vi "1_Face_Detection_Model_Converter.vi"() -> ()   [LabVIEW 2020]
doc: "This example demonstrates the preparation process of pretrained Face Detection model to be deployed on FPGA.\nIt consists of the following stages:\n1. Network optimization by merging applicable layers together.\n2. Per layer weights and output statistics calculation for optimal quantization on FPGA.\n3. Saving converted model together with statistical information to be used during the deployment.\n\nMore Examples: https://github.com/ngenehub/deepltk_fpga_examples"
uses:
  <vilib>/Ngene/DeepLTK FPGA Addon/Toolkit/NNF_Host/Low_Level/Network_Converter/Controls/Range_Calculation_Specs.ctl
  <vilib>/Ngene/Deep Learning Toolkit/Toolkit/Deep_Learning_Toolkit_by_Ngene.lvlib
  <vilib>/Ngene/DeepLTK FPGA Addon/Toolkit/DeepLTK_FPGA_Addon.lvlib
panel:
  in  "Dataset Path (Images)":path
  out "error out":errorcluster
  in  "Wights file":path
  in  "Configuration file":path
  out "Generated_Files":path[](array[path])
  in  "Dest":path
  # "Overview: This example demonstrates the preparation process of pretrained Face Detection model to be deployed on FPGA.\nIt consists of the following stages:\n1. Network optimization by merging applicable layers together.\n2. Per layer weights and output statistics calculation for optimal quantization on FPGA.\n3. Saving converted model together with statistical information to be used during the deployment.\nRequirements:\n•DeepLTK - Deep Learning Toolkit for LabVIEW\n•DeepLTK FPGA Addon\n•Sample dataset for reliable output statistic calculation.\n•NI Vision Development Module\nInstructions: \nNote: This VI can run as is by automatically retrieving required files from the example. I.e. steps 1. - 2. are optional.\n1.\tProvide the path to the configuration file of a pretrained model in the \"Configuration File\" control.\n2.\tProvide the path to the weights file of a pretrained model in the \"Weights File\" control. \n3.\tProvide the path to the WIDER FACE dataset images in the \"Dataset Path (Images)\" control. Dataset link: http://shuoyang1213.me/WIDERFACE/ \n4.\tProvide the destination directory where the result will be stored in the \"Dest\" control.\n5.\tRun the VI and wait until all processes are completed.\n\nThe resulting files (Scalers .cfg, Weights .bin, and Configuration .cfg) will be stored at paths displayed in \"Generated_Files\" indicator.\nThis files will be used during inference process.\nMore Examples: https://github.com/ngenehub/deepltk_fpga_examples"
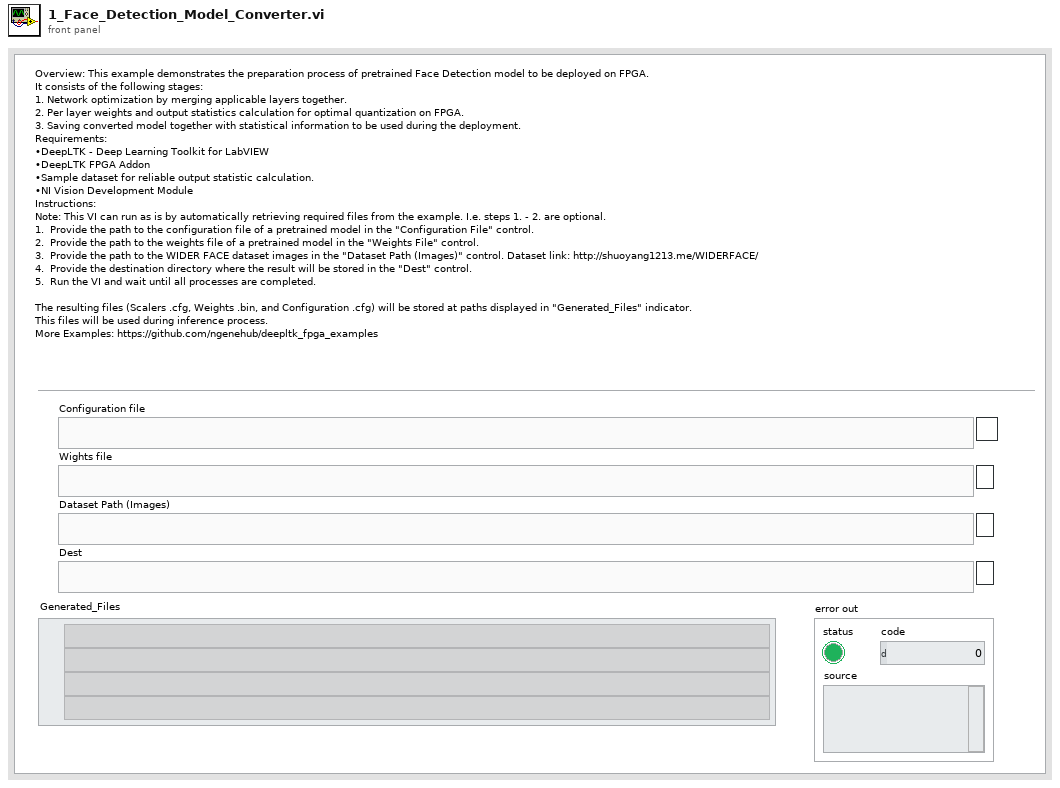
[diagram p1: front panel]
types:
  T1 = typedef "DeepLTK_FPGA_Addon.lvlib/Range_Calculation_Specs.ctl" = cluster{"# of Histogram Bins":i32, "Outputs Range Percentile(0.9999)":dbl, "Weights Range Percentile(0.9999)":dbl}
  T2 = typedef "Deep_Learning_Toolkit_by_Ngene.lvlib/NN_DataSet(In3D_OutBBox).ctl" = cluster{"Inputs Ref.":variant, "Dataset_Size":i32, "Dims_In":T3, "Outputs Refs":T4, "No of Classes ":i32, "Labels":string[], "File Paths":path[]}
  T3 = typedef "Deep_Learning_Toolkit_by_Ngene.lvlib/NN_Dims(C,H,W).ctl" = cluster{"C":i32, "H":i32, "W":i32}
  T4 = typedef "Deep_Learning_Toolkit_by_Ngene.lvlib/NN_Data_ref(1D_BBox).ctl" = refnum<data-value>
  T5 = typedef "Deep_Learning_Toolkit_by_Ngene.lvlib/NN_Config_Params.ctl" = cluster{"Name":string, "mBatch":i32, "NN_Train_Params":T6, "LR_Decay_Policy":T9, "Labels":string[], "Loss":T11}
  T6 = typedef "Deep_Learning_Toolkit_by_Ngene.lvlib/NN_Train_Params.ctl" = cluster{"Optimizer":T7, "Beta_1":sgl, "Beta_2":sgl, "Weight Decay(L1)":sgl, "Weight Decay(L2)":sgl, "Data_Sampling":T8}
  T7 = typedef "Deep_Learning_Toolkit_by_Ngene.lvlib/NN_Train_Optimizer.ctl" = enum16{"SGD", "Adam", "Adagrad", "Adadelta", "RMSProp", "Nesterov"}
  T8 = typedef "Deep_Learning_Toolkit_by_Ngene.lvlib/NN_Train_Data_Sampling.ctl" = enum16{"Random", "Sequential"}
  T9 = typedef "Deep_Learning_Toolkit_by_Ngene.lvlib/NN_LR_Policy_Cfg.ctl" = cluster{"Policy_Type":T10, "LR0":dbl, "k":sgl, "WarmUp_Policy":enum16{"Step", "Ramp"}, "WarmUp_Iter":i32, "WarmUp_Ratio":sgl}
  T10 = typedef "Deep_Learning_Toolkit_by_Ngene.lvlib/NN_LR_Policy_Type.ctl" = enum16{"Manual", "Step", "Exp", "1/t"}
  T11 = typedef "Deep_Learning_Toolkit_by_Ngene.lvlib/NN_Loss_Config_Params.ctl" = cluster{"Loss_Type":T12, "Loss_Conf_Params":variant}
  T12 = typedef "Deep_Learning_Toolkit_by_Ngene.lvlib/NN_Loss_Type.ctl" = enum16{"None", "MSE", "CrossEntropy", "YOLO_v2", "YOLO_v4"}
  T13 = typedef "Deep_Learning_Toolkit_by_Ngene.lvlib/NN_Layer_Config_Params.ctl" = cluster{"Layer_Type":T14, "Layer_Conf_Params":variant, "Input Layers":string[]}
  T14 = typedef "Deep_Learning_Toolkit_by_Ngene.lvlib/NN_Layer_Type.ctl" = enum16{"Input1D", "Input3D", "Conv1D", "Conv2D", "Conv2D_Adv", "MaxPool", "AvgPool", "UpSample", "DropOut3D", "ShortCut", "Concat", "SoftMax3D", "FC", "DropOut", "Softmax", "Flatten", "YOLO_v2", "YOLO_v4", "Activation", "BatchNormalization", "Unsupported"}
  T15 = typedef "Deep_Learning_Toolkit_by_Ngene.lvlib/NN.ctl" = cluster{"Name":string, "No of Layers":i32, "mBatch":i32, "Layers":T16[], "Dimty":T17, "Dims_In":T3, "Dims_Out":T3, "Working_Dir":path, "Train?":bool, "Train_Params":T6, "LR_Update_Policy":T9, "Session Data":T18, "Ground_truth":T19, "NNg_hdls":T20, "NN_Device":T21, "GPU Id":i32, "Labels":string[], "Receptive Field":T22[], "Loss_Type":T12, "Loss_Cfg_Prms":variant, "NNG_WS":T23}
  T16 = typedef "Deep_Learning_Toolkit_by_Ngene.lvlib/NN_Layer_ref.ctl" = refnum<data-value>
  T17 = typedef "Deep_Learning_Toolkit_by_Ngene.lvlib/NN_In_Out_Dim-ty.ctl" = enum8{"In1D_Out1D", "In3D_Out1D", "In3D_Out3D", "In3D_OutBBox"}
  T18 = typedef "Deep_Learning_Toolkit_by_Ngene.lvlib/NN_Train_Session_Data.ctl" = cluster{"Epochs":sgl, "Tot_Iter":i32, "LR":sgl, "LR_iter":i32}
  T19 = typedef "Deep_Learning_Toolkit_by_Ngene.lvlib/NN_Ground_truth.ctl" = cluster{"Y":variant}
  T20 = typedef "Deep_Learning_Toolkit_by_Ngene.lvlib/nng_cuda_handles.ctl" = cluster{"cudnn":u64, "cublas":u64, "stream":u64, "curand":u64}
  T21 = typedef "Deep_Learning_Toolkit_by_Ngene.lvlib/NN_Device.ctl" = enum16{"CPU", "GPU"}
  T22 = typedef "Deep_Learning_Toolkit_by_Ngene.lvlib/NN_Dims(V,H).ctl" = cluster{"V":i32, "H":i32}
  T23 = typedef "Deep_Learning_Toolkit_by_Ngene.lvlib/NNG_WS.ctl" = cluster{"NNG_WS_Mem":T24, "Max_WS_Size":i64}
  T24 = typedef "Deep_Learning_Toolkit_by_Ngene.lvlib/NNg_WS_Mem_DVR.ctl" = refnum<data-value>
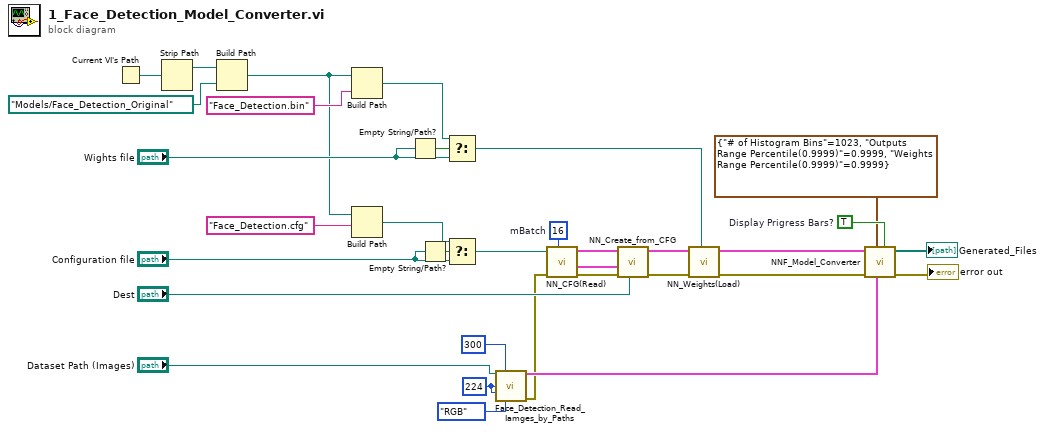
[diagram p0: block diagram]
diagram:
  w14 = 224 ("Img Height")
  w23 = TRUE  # Display Prigress Bars?
  w27 = 16  # mBatch
  n1 = Current VI's Path() -> (path=w4:path)
  n2 = Strip Path(path=w4) -> (stripped path=w6:path)  [unwired: 1 out]
  n3 = Build Path(base path=w6, name or relative path=path "Models/Face_Detection_Original" ("stripped path")) -> (appended path=w3:path)
  n4 = Build Path(base path=w3, name or relative path="Face_Detection.bin") -> (appended path=w2:path)
  n5 = Build Path(base path=w3, name or relative path="Face_Detection.cfg") -> (appended path=w1:path)
  n6 = Empty String/Path?(string/path="Wights file") -> (empty?=w15:bool)
  n7 = Empty String/Path?(string/path="Configuration file") -> (empty?=w16:bool)
  n8 = Select(t=w2, s=w15, f="Wights file") -> (s? t:f=w19:path)
  n9 = Select(t=w1, s=w16, f="Configuration file") -> (s? t:f=w20:path)
  n10 = call "Face_Detection_Read_Iamges_by_Paths.vi"("Dataset Path (Images)"="Dataset Path (Images)", "Max Sample count"=300, "Img Height"=w14, "Img Width"=w14, "Img Type"=enum16{"Grayscale", "RGB"}."RGB") -> ("NN_DataSet(In3D_OutBBox)"=w11:T2, "error out"=w10:errorcluster)  [unwired: 9 in]
  n11 = call <vilib>:"NN_CFG(Read).vi"("mBatch"=w27, "error in (no error)"=w10, "CFG file path"=w20) -> ("error out"=w30:errorcluster, "Net_Cfg"=w33:T5, "Layer_Cfg"=w29:T13[])  [unwired: 6 in]
  n12 = call <vilib>:"NN_Create_from_CFG.vi"("Working Dir"="Dest", "error in (no error)"=w30, "Net_Cfg"=w33, "Layer_Cfg"=w29) -> ("error out"=w31:errorcluster, "NN out"=w32:T15)  [unwired: 6 in]
  n13 = call <vilib>:"NN_Weights(Load).vi"("Weight File Path"=w19, "error in (no error)"=w31, "NN in"=w32) -> ("error out"=w28:errorcluster, "NN out"=w24:T15)  [unwired: 7 in]
  n14 = call <vilib>:"NNF_Model_Converter.vi"("Display Progress Bars?"=w23, "DataSet"=w11, "Range_Calculation_Specs"=T1 {"# of Histogram Bins"=1023, "Outputs Range Percentile(0.9999)"=0.9999, "Weights Range Percentile(0.9999)"=0.9999}, "error in (no error)"=w28, "NN in"=w24) -> ("error out"=→"error out":errorcluster, "Generated_Files"=→"Generated_Files":path[])  [unwired: 3 in, 2 out]
